vi "ToJson.vi"(8 "error in (no error)":errorcluster, 11 "Room in":refnum<class "Room.lvclass">) -> (0 "error out":errorcluster, 2 "String":string, 3 "Room out":refnum<class "Room.lvclass">)   [LabVIEW 2015, in "Room.lvclass"]
uses:
  Room.lvclass
  JsonCluster.ctl
  Room.lvclass/Room.ctl
  Flags/Flags.lvclass/Flags.ctl
  Flags/Read Color.vi
  Flags/Read State.vi
  Flags/Flags.lvclass
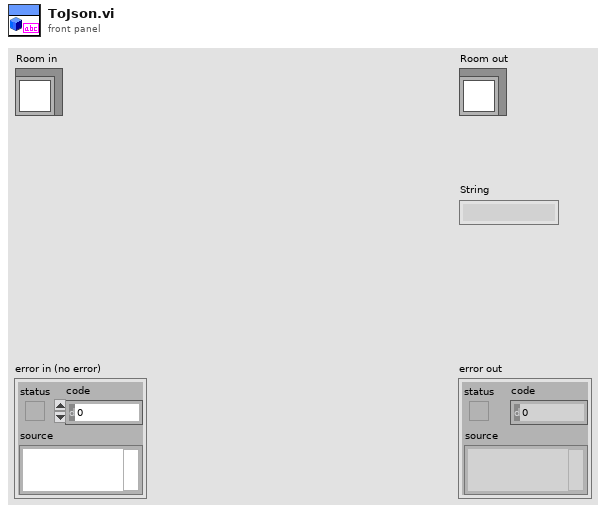
[diagram p1: front panel]
types:
  T1 = typedef "Room.lvclass/JsonCluster.ctl" = cluster{"Flags":cluster{"State":bool[], "Color":i32[]}, "BedVacant":bool, "InRoomPersonnel":string[], "RoomRequests":string[], "BeaconId":string, "BedURL":string, "RoomNumber":i32}
  T2 = typedef "Flags.lvclass/ColorEnum.ctl" = enum8{"Red", "Blue", "Green", "Yellow"}
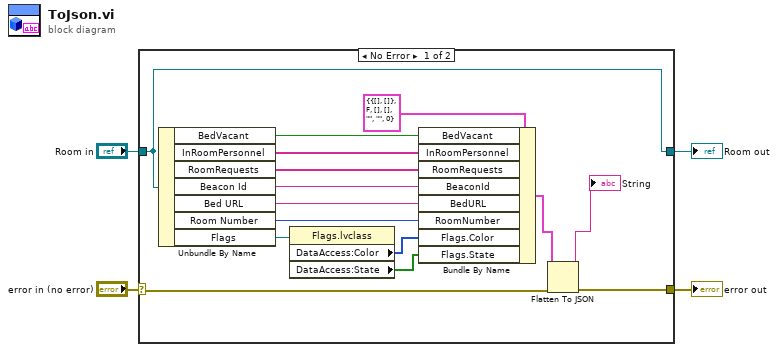
[diagram p0: block diagram]
diagram:
  n1 = case shown="No Error" "error in (no error)" {
    selector: "error in (no error)" -> [w5 w21]
    tunnel: [w15 w21] -> w3
    tunnel: [w19 w20] -> w1
    tunnel: "Room in" -> [w19 w20]
    frame No Error {
      n2 = Unbundle By Name(w19) -> ("BedVacant"=w14:bool, "InRoomPersonnel"=w13:string[], "RoomRequests"=w12:string[], "Beacon Id"=w11:string, "Bed URL"=w10:string, "Room Number"=w9:i32, "Flags"=w8:refnum<class "Flags.lvclass">)
      n3 = property class="Flags.lvclass"(reference=w8) -> ("DataAccess:Color"=w7:T2[], "DataAccess:State"=w6:bool[])  [unwired: 1 in, 2 out]
      n4 = Bundle By Name(cluster=T1 {"Flags"={"State"=[], "Color"=[]}, "BedVacant"=FALSE, "InRoomPersonnel"=[], "RoomRequests"=[], "BeaconId"="", "BedURL"="", "RoomNumber"=0} ("Room"), "BedVacant"=w14, "InRoomPersonnel"=w13, "RoomRequests"=w12, "BeaconId"=w11, "BedURL"=w10, "RoomNumber"=w9, "Flags.Color"=w7, "Flags.State"=w6) -> (w16:T1)
      n5 = Flatten To JSON(anything=w16, error in (no error)=w5) -> (JSON string=→"String":string, 11:w15:errorcluster)  [unwired: 1 in]
    }
    frame Error {
    }
  }
  "error out" <- w3
  "Room out" <- w1
